vi "To Close Session Behavior.vi"(11 "initialize and close session behavior":T2) -> (3 "close session behavior":T1)   [LabVIEW 2020, in "MeasurementLink Instrument.lvlib" / "IInstrument.lvclass"]
uses:
  IInstrument.lvclass
  Initialize and Close Session Behavior.ctl
  Close Session Behavior.ctl
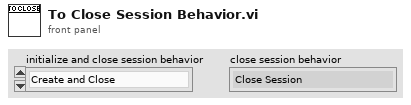
[diagram p1: front panel]
types:
  T1 = typedef "MeasurementLink Instrument.lvlib/IInstrument.lvclass/Close Session Behavior.ctl" = enum16{"Close Session", "Detach Session"}
  T2 = typedef "MeasurementLink Instrument.lvlib/IInstrument.lvclass/Initialize and Close Session Behavior.ctl" = enum16{"Create and Close", "Attach and Detach", "Create and Detach", "Attach and Close"}
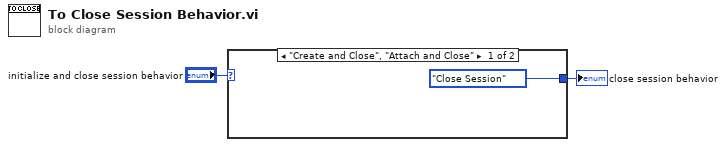
[diagram p0: block diagram]
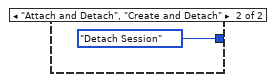
[diagram p2: hidden frame]
diagram:
  n1 = case shown="\"Create and Close\", \"Attach and Close\"" "initialize and close session behavior" {
    tunnel: [Close_Session_Behavior."Close Session" ("close session behavior") Close_Session_Behavior."Detach Session" ("close session behavior")] -> w1
    frame "Create and Close", "Attach and Close" {
    }
    frame "Attach and Detach", "Create and Detach" {
    }
  }
  "close session behavior" <- w1
